vi "DB UI - Search-Load Setup.vi"(11 "Refnums":T4) -> (0 "Error Out":errorcluster, 1 "{Cancel}":bool, 2 "Transaction":T3, 3 "1D Results":string[](array[string]))   [LabVIEW 2013]
uses:
  Controls/Combo Box.ctl
  Controls/DB - Refnums.ctl
  Controls/Setup - Part Details - Item Details.ctl
  <vilib>/Utility/miscctls.llb/LVRectTypeDef.ctl
  Controls/Transaction Cluster.ctl
  Controls/Debug Tab.ctl
  <vilib>/Utility/miscctls.llb/LVRowAndColumnUnsignedTypeDef.ctl
  <vilib>/Utility/miscctls.llb/LVPointTypeDef.ctl
  <vilib>/Utility/miscctls.llb/LVRowAndColumnTypeDef.ctl
  Controls/DB - Setup Item Enum.ctl
panel:
  in  "OR [CaptionOnly]":string caption="OR"
  in  "Tab Control":T1
  out "Get Clicked Column Header":i32
  in  "Ascending":bool
  out "Time":u32
  out "x":u32
  out "y":u32
  out "Front Panel Window:Panel Bounds":T2
  out "2D Results":string[][](array[string])=[["Production", "OperationNo1"], ["Production", "Qty1"], ["Production", "NCRNo1"], ["Production", "CustomerID1"], ["Production", "Customer1"], ["Production", "Project1"], ["Production", "SalesOrderNo1"], ["Production", "SalesOrderItemNo1"], ["Production", "MaterialNo1"], ["Production", "MaterialRev1"], ["Production", "MaterialDesc1"], ["Production", "SerialNos1"], ["Production", "UnitOfQty1"]]
  out "Drop Down":bool
  in  "CellBG New Cells":u32(colorbox)=16777225
  in  "CellBG Unused Cells":u32(colorbox)=16777238
  in  "CellBG ColHdrs":u32(colorbox)=11776947
  out "MHandler Error":errorcluster
  in  "Criteria [CaptionOnly]":string caption="Criteria"
  in  "Cancel":bool caption="Report Execute Search"
  in  "Open":bool caption="Report Execute Search"
  in  "Search":bool caption="Report Execute Search"
  in  "Report List":i32(listbox)=-1 caption="List"
  in  "OrderNo":T5 caption="Order No."
  in  "TransactionNo":T5 caption="Transaction No."
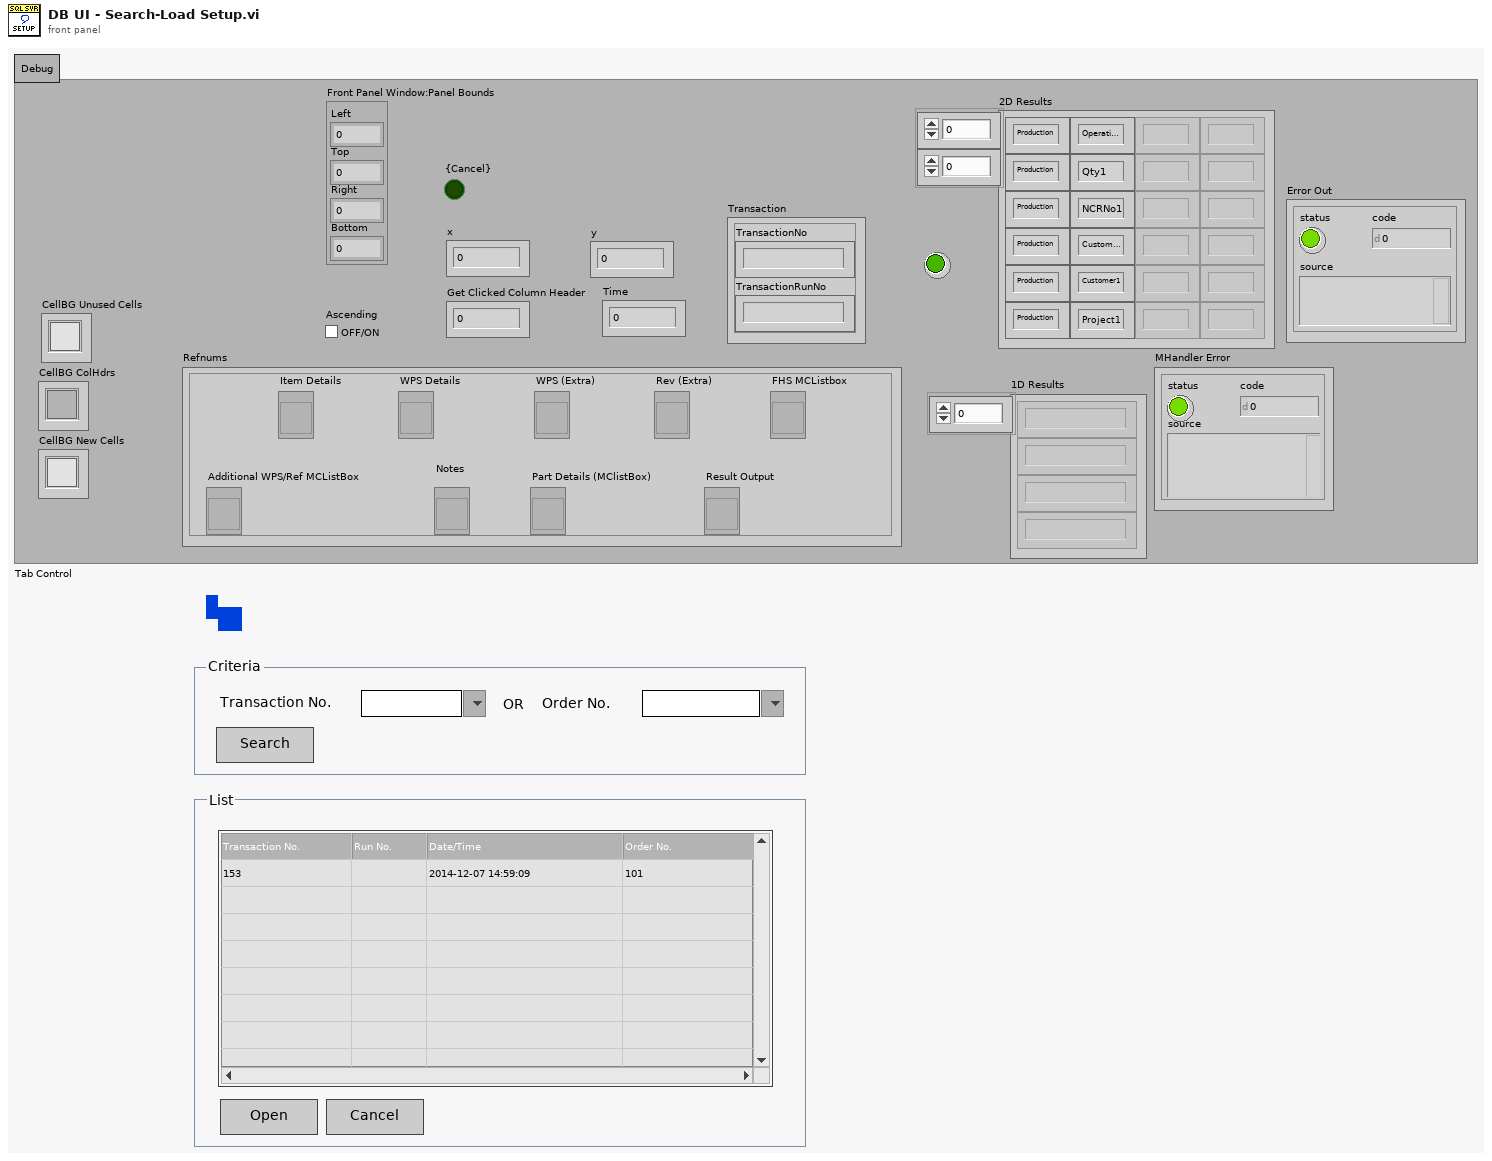
[diagram p1: front panel]
types:
  T1 = typedef "Debug Tab.ctl" = enum32{"Debug"}
  T2 = typedef "LVRectTypeDef.ctl" = cluster{"Left":i16, "Top":i16, "Right":i16, "Bottom":i16}
  T3 = typedef "Transaction Cluster.ctl" = cluster{"TransactionNo":string, "TransactionRunNo":string}
  T4 = typedef "DB - Refnums.ctl" = cluster{"Item Details":refnum<vi>, "WPS Details":refnum<vi>, "WPS (Extra)":refnum<vi>, "Rev (Extra) ":refnum<vi>, "FHS MCListbox":refnum<vi>, "Additional WPS/Ref MCListBox":refnum<vi>, "Notes":refnum<vi>, "Part Details (MClistBox)":refnum<vi>, "Result Output":refnum<vi>}
  T5 = typedef "Combo Box.ctl" = string
  T6 = typedef "LVPointTypeDef.ctl" = cluster{"Horizontal":i16, "Vertical":i16}
  T7 = typedef "LVRowAndColumnUnsignedTypeDef.ctl" = cluster{"Row":u32, "Column":u32}
  T8 = typedef "LVRowAndColumnTypeDef.ctl" = cluster{"Row":i32, "Column":i32}
  T9 = typedef "DB - Setup Item Enum.ctl" = enum16{"SELECT [Plant],[OrderNo]", "INSERT [Setup].[Header]", "INSERT [Setup].[Item]", "INSERT [Setup].[ProcedureItem]", "SELECT [TransactionNo]", "SELECT [TransactionNo], others", "SELECT [OrderNo]", "SELECT [OrderNo], others", "SELECT h.[TransactionNo], i.[OrderNo]", "SELECT [Setup].[ProcedureItem]", "SELECT [EquipmentxId]"}
  T10 = enum8{"Enabled", "Disabled", "Disabled and Grayed Out"}
  T11 = cluster{"TransactionNo":string, "TransactionRunNo":string}
  T12 = typedef "eventvkey.ctl" = enum16{"ASCII", "Enter", "Return", "Shift", "Ctrl", "Alt", "Cmd", "Opt", "Caps", "NumLock", "Clear", "Break", "Up", "Down", "Left", "Right", "Insert", "Delete", "Home", "End", "PageUp", "PageDown", "Escape", "Help", "Pause", "ScrollLock", "F1", "F2", "F3", "F4", "F5", "F6", "F7", "F8", "F9", "F10", "F11", "F12", "F13", "F14", "F15", "F16", "F17", "F18", "F19", "F20", "F21", "F22", "F23", "F24", "Play", "VolumeUp", "VolumeDown", "Mute", "Two Byte Char"}
  T13 = typedef "LVPoint32TypeDef.ctl" = cluster{"Horizontal":i32, "Vertical":i32}
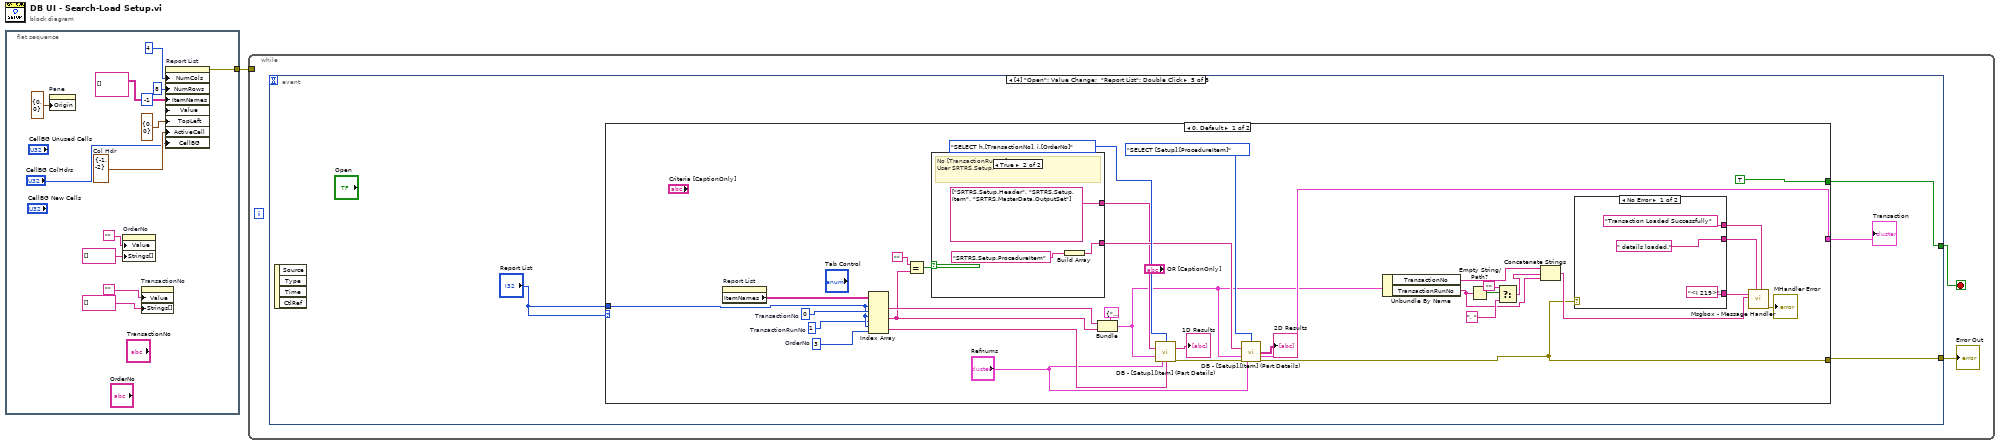
[diagram p0: block diagram]
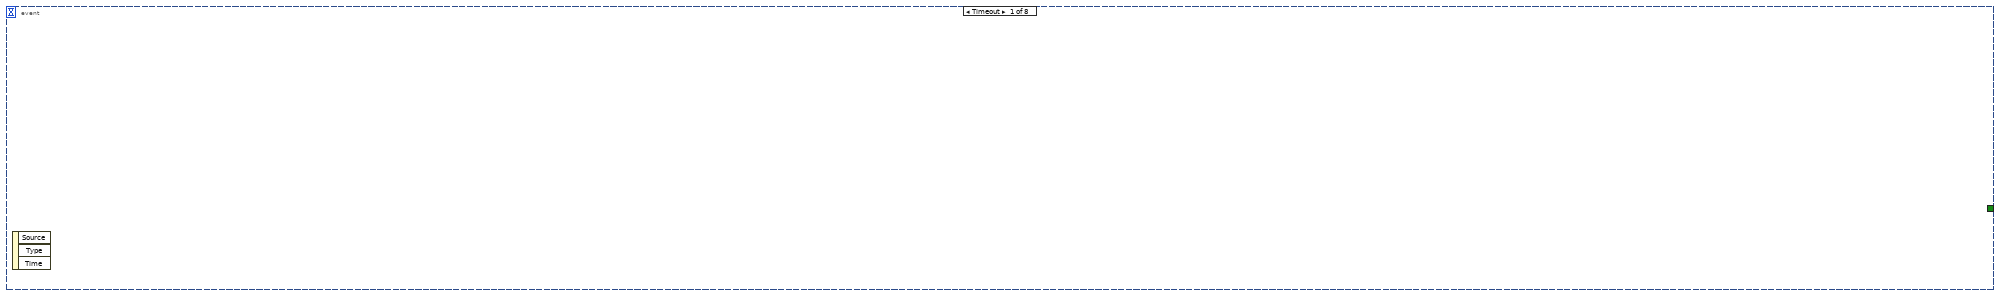
[diagram p2: hidden frame]
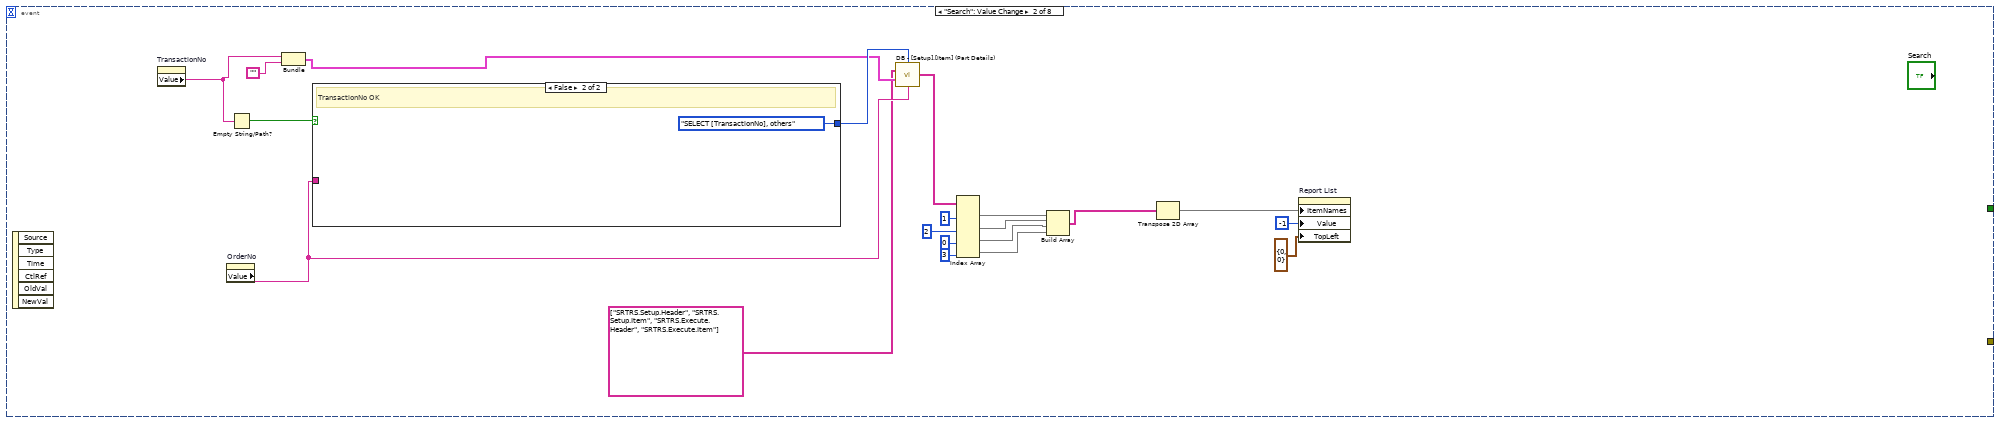
[diagram p3: hidden frame]
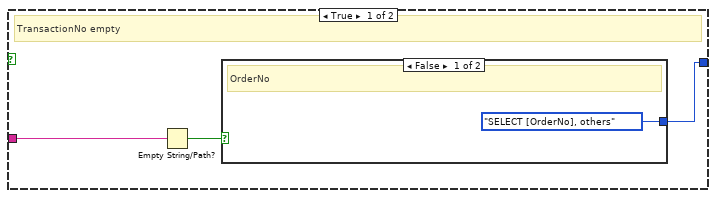
[diagram p4: hidden frame]
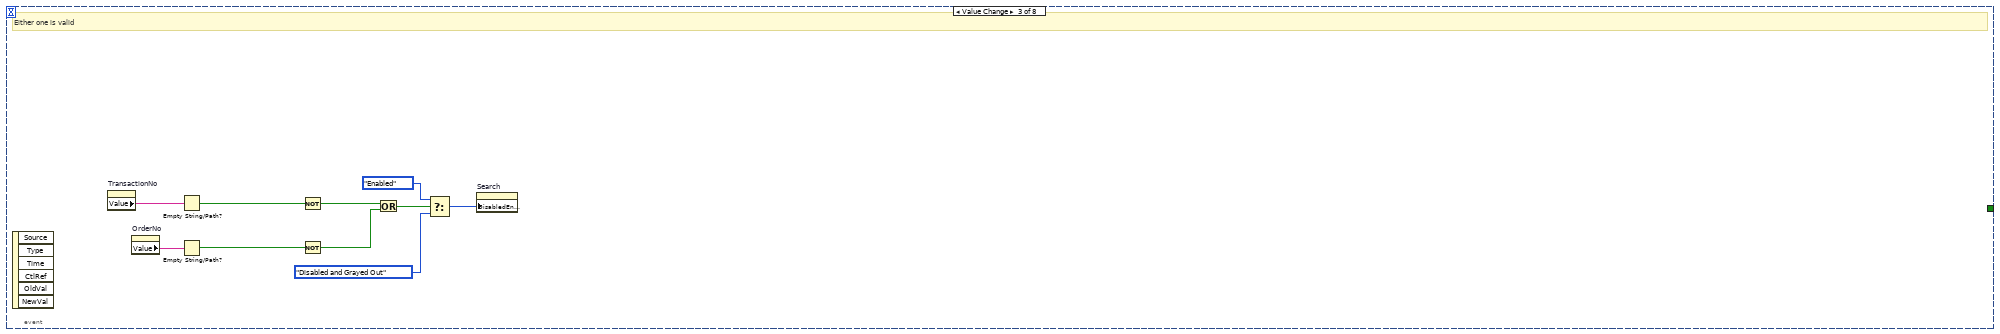
[diagram p6: hidden frame]
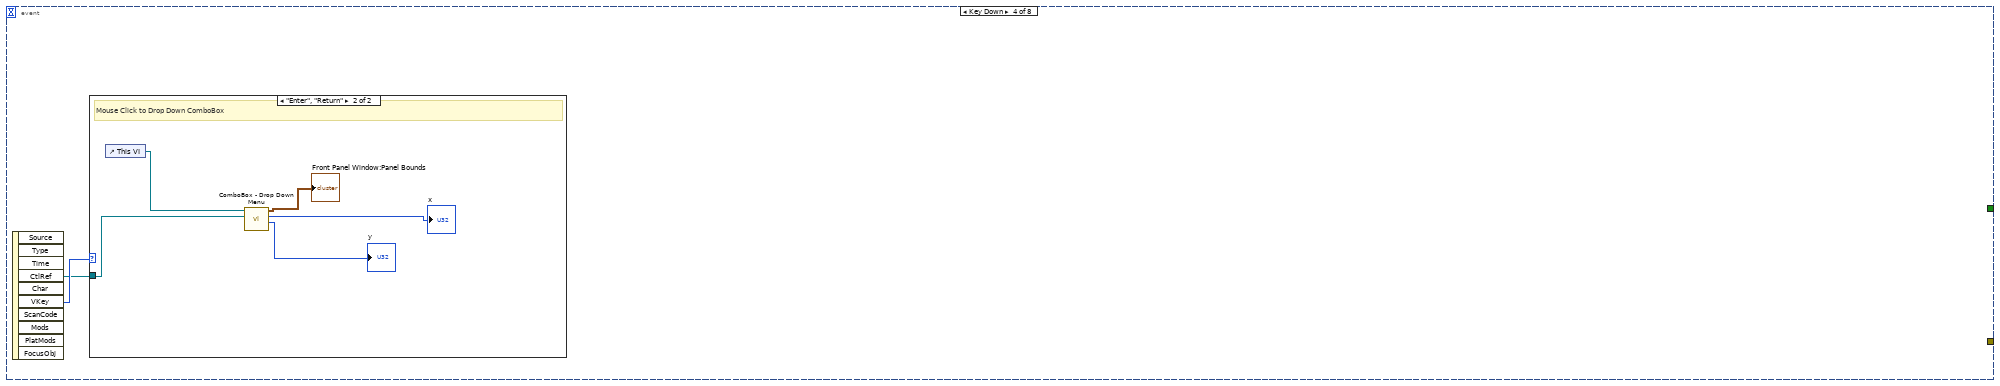
[diagram p7: hidden frame]
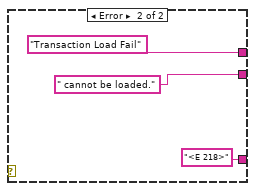
[diagram p9: hidden frame]
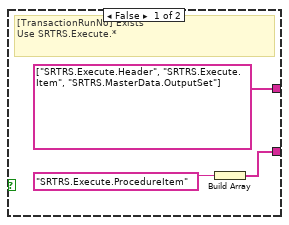
[diagram p10: hidden frame]
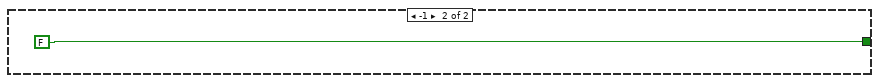
[diagram p11: hidden frame]
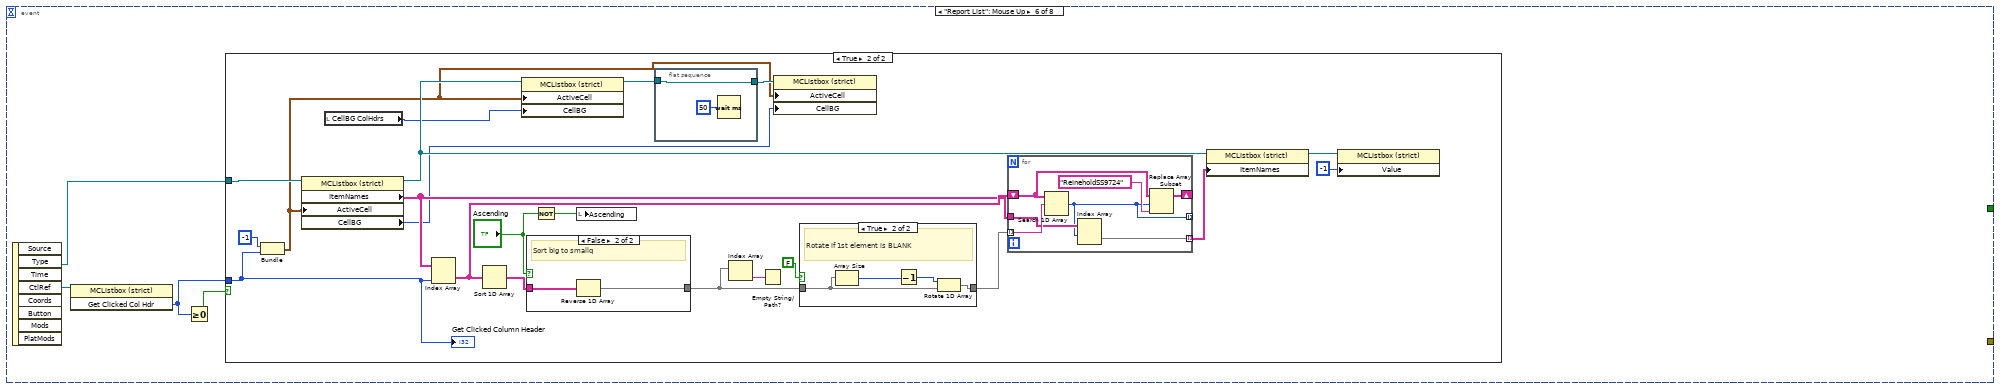
[diagram p12: hidden frame]
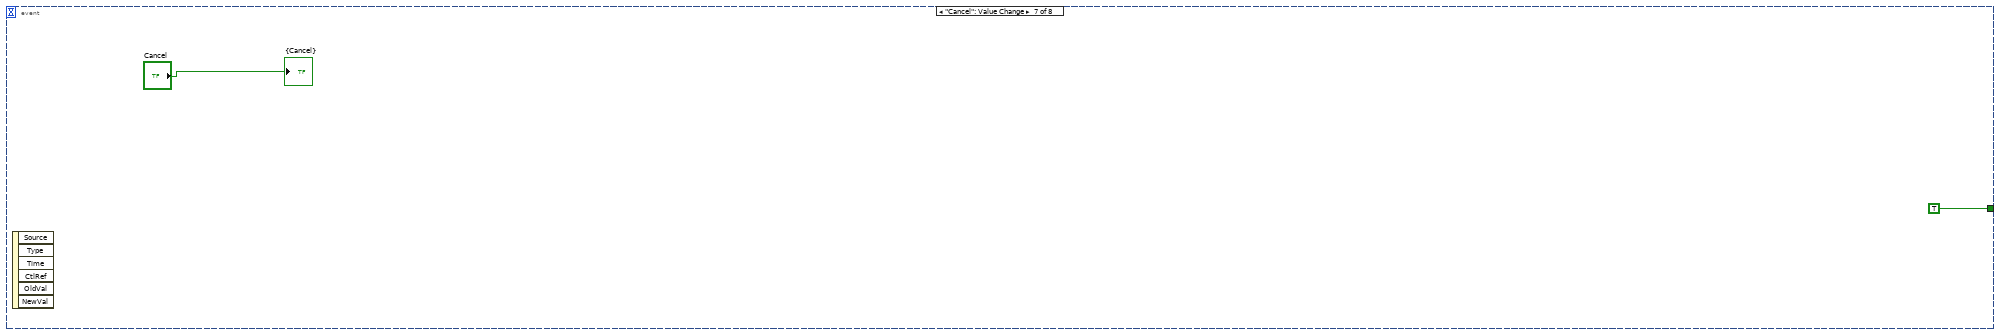
[diagram p16: hidden frame]
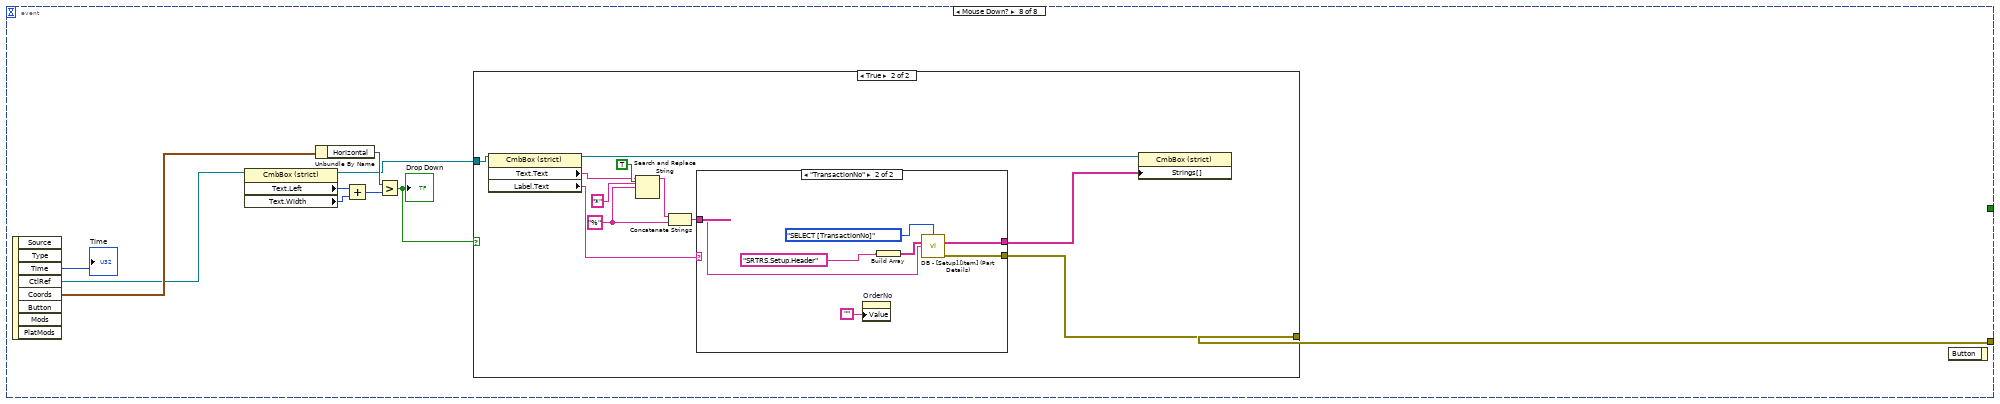
[diagram p17: hidden frame]
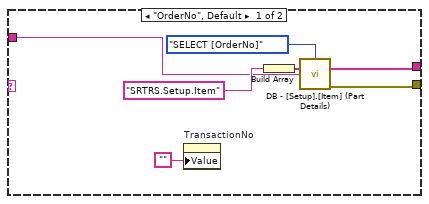
[diagram p19: hidden frame]
diagram:
  n1 = flat-sequence {
    tunnel: [w13] -> w1
    frame #0 {
      w3 = T8 {"Row"=-1, "Column"=-2}  # Col Hdr
      n2 = property on="Pane" class="Pane"("Origin"=T6 {"Horizontal"=0, "Vertical"=0}) -> ()  [unwired: 2 in, 2 out]
      n3 = property on="OrderNo" class="CmbBox (strict)"("Value"="", "Strings[]"=string[] [] ("Strings []")) -> ()  [unwired: 2 in, 2 out]
      n4 = property on="TransactionNo" class="CmbBox (strict)"("Value"="", "Strings[]"=string[] [] ("Strings []")) -> ()  [unwired: 2 in, 2 out]
      n5 = property on="Report List" class="MCListbox (strict)"("NumCols"=u32 4 ("Number of Columns"), "NumRows"=u32 8 ("Number of Rows"), "ItemNames"=string[][] [] ("Item Names"), "Value"=-1 ("Report List"), "TopLeft"=T7 {"Row"=0, "Column"=0} ("Top Left Visible Cell"), "ActiveCell"=w3, "CellBG"="CellBG ColHdrs") -> (error out=w13:errorcluster)  [unwired: 2 in, 1 out]
    }
  }
  n6 = while {
    tunnel: w1 -> [_]
    stop <- w16 stop-if-true
    n7 = event shown="[4] \"Open\": Value Change;  \"Report List\": Double Click" {
      selector: _ -> [_ _ _ _ _ _ _ _]
      dyn-events: _ -> [_ _ _ _ _ _ _ _]
      timeout: _ -> [_ _ _ _ _ _ _ _]
      tunnel: [_ _ _ _ w61 _ TRUE ("Cancel") _] -> w16
      tunnel: [_ _ _ _ w59 _ _ w162] -> w15
      event Timeout {
        n8 = event-data() -> ()  [unwired: 1 in, 3 out]
      }
      event "Search": Value Change {
        n9 = event-data() -> ()  [unwired: 1 in, 6 out]
        n10 = property on="TransactionNo" class="CmbBox (strict)"() -> ("Value"=w20:T5)  [unwired: 2 in, 2 out]
        n11 = property on="OrderNo" class="CmbBox (strict)"() -> ("Value"=w34:T5)  [unwired: 2 in, 2 out]
        n12 = Empty String/Path?(string/path=w20) -> (empty?=w36:bool)
        n13 = Bundle("Value"=w20, "") -> (w19:cluster{"Value":T5, string})  [unwired: 1 in]
        n14 = case shown="False" w36 {
          tunnel: w34 -> [w39 _]
          tunnel: [w37 DB_-_Setup_Item_Enum."SELECT [TransactionNo], others" ("DB - Setup Item Enum")] -> w35
          frame True {
            # "TransactionNo empty"
            n15 = Empty String/Path?(string/path=w39) -> (empty?=w38:bool)
            n16 = case shown="False" w38 {
              tunnel: [DB_-_Setup_Item_Enum."SELECT [OrderNo], others" ("DB - Setup Item Enum") _] -> w37
              frame False {
                # "OrderNo"
              }
              frame True {
                # "OrderNo empty"
              }
            }
          }
          frame False {
            # "TransactionNo OK"
          }
        }
        n17 = call "DB - [Setup].[Item] (Part Details).vi"("DB - Setup Item Enum"=w35, "DB.Schema.Table Array"=string[] ["SRTRS.Setup.Header", "SRTRS.Setup.Item", "SRTRS.Execute.Header", "SRTRS.Execute.Item"], "Transaction"=w19, "OrderNo"=w34) -> ("2D Results"=w31:string[][])  [unwired: 6 in, 5 out]
        n18 = Index Array(array=w31, index (col) #1=1 ("disabled index (col)"), index (col) #2=2 ("index (col)"), index (col) #3=0 ("index (col)"), index (col) #4=3 ("index (col)")) -> (element #1=w29:string[], element #2=w27:string[], element #3=w25:string[], element #4=w24:string[])  [unwired: 4 in]
        n19 = Build Array(w29, w27, w25, w24) -> (w23:string[][])
        n20 = Transpose 2D Array(2D array=w23) -> (transposed array=w22:string[][])
        n21 = property on="Report List" class="MCListbox (strict)"("ItemNames"=w22, "Value"=-1 ("Report List"), "TopLeft"=T7 {"Row"=0, "Column"=0} ("Top Left Visible Cell")) -> ()  [unwired: 2 in, 2 out]
      }
      event Value Change {
        # "Either one is valid"
        n22 = event-data() -> ()  [unwired: 1 in, 6 out]
        n23 = property on="TransactionNo" class="CmbBox (strict)"() -> ("Value"=w51:T5)  [unwired: 2 in, 2 out]
        n24 = property on="OrderNo" class="CmbBox (strict)"() -> ("Value"=w50:T5)  [unwired: 2 in, 2 out]
        n25 = Empty String/Path?(string/path=w51) -> (empty?=w49:bool)
        n26 = Empty String/Path?(string/path=w50) -> (empty?=w48:bool)
        n27 = Not(x=w49) -> (.not. x?=w47:bool)
        n28 = Not(x=w48) -> (.not. x?=w46:bool)
        n29 = Or(x=w47, y=w46) -> (x .or. y?=w45:bool)
        n30 = Select(t=T10."Enabled" ("Disabled"), s=w45, f=T10."Disabled and Grayed Out" ("Disabled")) -> (s? t:f=w43:T10)
        n31 = property on="Search" class="Bool"("DisabledEnum"=w43) -> ()  [unwired: 2 in, 2 out]
      }
      event Key Down {
        n32 = event-data() -> ("CtlRef"=w52:refnum<vi>, "VKey"=w53:T12)  [unwired: 1 in, 8 out]
        n33 = case shown="\"Enter\", \"Return\"" w53 {
          tunnel: w52 -> [_ w57]
          frame "ASCII", Default {
          }
          frame "Enter", "Return" {
            # "Mouse Click to Drop Down ComboBox"
            n34 = control-ref of="This VI"() -> (w58:refnum<vi>)
            n35 = call "ComboBox - Drop Down Menu.vi"("CtlRef"=w57, "VI in (This VI)"=w58) -> ("y"=→"y":u32, "x"=→"x":u32, "Front Panel Window:Panel Bounds"=→"Front Panel Window:Panel Bounds":T2)  [unwired: 7 in]
          }
        }
      }
      event "Open": Value Change; "Report List": Double Click {
        n36 = event-data() -> ()  [unwired: 1 in, 4 out]
        n37 = case shown="0, Default" "Report List" {
          tunnel: "Report List" -> [w86 _]
          tunnel: [w64 _] -> w59
          tunnel: [TRUE ("Cancel") FALSE ("Cancel")] -> w61
          tunnel: [w84 _] -> w60
          frame 0, Default {
            w85 = 1  # TransactionRunNo
            w88 = 3  # OrderNo
            w95 = 0  # TransactionNo
            n38 = property on="Report List" class="MCListbox (strict)"() -> ("ItemNames"=w96:string[][])  [unwired: 2 in, 2 out]
            n39 = Index Array(array=w96, index (row) #1=w86, index (col) #1=w95, index (row) #2=w86, index (col) #2=w85, index (row) #3=w86, index (col) #3=w88) -> (element #1=w89:string, element #2=w83:string, element #3=w87:string)
            n40 = Equal?(x="", y=w83) -> (x = y?=w81:bool)
            n41 = case shown="True" w81 {
              tunnel: [w104 w106] -> w79
              tunnel: [string[] ["SRTRS.Execute.Header", "SRTRS.Execute.Item", "SRTRS.MasterData.OutputSet"] string[] ["SRTRS.Setup.Header", "SRTRS.Setup.Item", "SRTRS.MasterData.OutputSet"]] -> w78
              frame False {
                # "[TransactionRunNo] Exists\nUse SRTRS.Execute.*"
                n42 = Build Array("SRTRS.Execute.ProcedureItem" ("DB.Schema.Table")) -> (w104:string[])
              }
              frame True {
                # "No [TransactionRunNo]\nUser SRTRS.Setup.*"
                n43 = Build Array("SRTRS.Setup.ProcedureItem" ("DB.Schema.Table")) -> (w106:string[])
              }
            }
            n44 = Bundle(cluster=T11 {"TransactionNo"="", "TransactionRunNo"=""} ("output cluster"), "TransactionNo"=w89, "TransactionRunNo"=w83) -> (w63:T11)
            n45 = call "DB - [Setup].[Item] (Part Details).vi"("DB - Setup Item Enum"=DB_-_Setup_Item_Enum."SELECT h.[TransactionNo], i.[OrderNo]", "DB.Schema.Table Array"=w78, "Transaction"=w63, "DB Refnums"="Refnums", "OrderNo"=w87) -> ("1D Results"=→"1D Results":string[], "SUMMARY"=w93:errorcluster)  [unwired: 5 in, 4 out]
            n46 = call "DB - [Setup].[Item] (Part Details).vi"("DB - Setup Item Enum"=DB_-_Setup_Item_Enum."SELECT [Setup].[ProcedureItem]", "DB.Schema.Table Array"=w79, "Transaction"=w63, "error in (no error)"=w93, "DB Refnums"="Refnums") -> ("2D Results"=→"2D Results":string[][], "Transaction"=w84:T3, "SUMMARY"=w64:errorcluster)  [unwired: 5 in, 3 out]
            n47 = Unbundle By Name(w63) -> ("TransactionNo"=w69:string, "TransactionRunNo"=w65:string)
            n48 = Empty String/Path?(string/path=w65) -> (empty?=w70:bool)
            n49 = Select(t="", s=w70, f=", ") -> (s? t:f=w66:string)
            n50 = Concatenate Strings(w69, w66, w65) -> (w72:string)
            n51 = case shown="No Error" w64 {
              tunnel: ["<I 219>" ("<.?....> Message Code") "<E 218>" ("<.?....> Message Code")] -> w75
              tunnel: ["Transaction Loaded Successfully" ("Short Description (When DB Not Available)") "Transaction Load Fail" ("Short Description (When DB Not Available)")] -> w74
              tunnel: [" details loaded." ("Description (When DB Not Available)") " cannot be loaded." ("Description (When DB Not Available)")] -> w73
              frame No Error {
              }
              frame Error {
              }
            }
            n52 = call "Msgbox - Message Handler.vi"("Short Description (When DB Not Available)"=w74, "Description (When DB Not Available)"=w73, "Pre-Description"=w72, "<.?....> Message Code"=w75) -> ("MHandler Error"=→"MHandler Error":errorcluster)  [unwired: 5 in, 2 out]
          }
          frame -1 {
          }
        }
        "Transaction" <- w60
      }
      event "Report List": Mouse Up {
        n53 = event-data() -> ("CtlRef"=w112:refnum<vi>)  [unwired: 1 in, 7 out]
        n54 = invoke class="MCListbox (strict)" method="Get Clicked Col Hdr"(reference=w112) -> ("Get Clicked Column Header"=w111:i32)  [unwired: 2 in, 2 out]
        n55 = Greater Or Equal To 0?(x=w111) -> (x >= 0?=w110:bool)
        n56 = case shown="True" w110 {
          tunnel: w112 -> [_ w126]
          tunnel: w111 -> [_ w119]
          frame False {
          }
          frame True {
            n57 = Bundle(-1, "Get Clicked Column Header"=w119) -> (w116:cluster{i32, "Get Clicked Column Header":i32})  [unwired: 1 in]
            n58 = property class="MCListbox (strict)"(reference=w126, "ActiveCell"=w116) -> (reference out=w121:refnum<vi>, "ItemNames"=w125:string[][], "CellBG"=w115:u32)  [unwired: 1 in, 1 out]
            n59 = local read "CellBG ColHdrs"() -> (w113:u32)
            n60 = Index Array(array=w125, index (col)=w119) -> (element=w129:string[])  [unwired: 1 in]
            n61 = Sort 1D Array(array=w129) -> (sorted array=w132:string[])
            n62 = property class="MCListbox (strict)"(reference=w121, "ActiveCell"=w116, "CellBG"=w113) -> (reference out=w118:refnum<vi>)  [unwired: 1 in, 1 out]
            n63 = case shown="False" "Ascending" {
              tunnel: w132 -> [w141 w143]
              tunnel: [w141 w142] -> w127
              frame True {
                # "Sort small to big p"
              }
              frame False {
                # "Sort big to smallq"
                n64 = Reverse 1D Array(array=w143) -> (reversed array=w142:string[])
              }
            }
            n65 = Not(x="Ascending") -> (.not. x?=w122:bool)
            n66 = local write "Ascending"(w122) -> ()
            n67 = flat-sequence {
              tunnel: w118 -> [w135]
              tunnel: [w135] -> w117
              frame #0 {
                n68 = Wait (ms)(milliseconds to wait=u32 50) -> ()  [unwired: 1 out]
              }
            }
            n69 = Index Array(array=w127) -> (element=w128:string)  [unwired: 1 in]
            n70 = Empty String/Path?(string/path=w128) -> ()  [unwired: 1 out]
            n71 = property class="MCListbox (strict)"(reference=w117, "ActiveCell"=w116, "CellBG"=w115) -> ()  [unwired: 1 in, 2 out]
            n72 = case shown="True" FALSE {
              tunnel: w127 -> [w136 w139]
              tunnel: [w136 w140] -> w124
              frame False {
              }
              frame True {
                # "Rotate if 1st element is BLANK"
                n73 = Array Size(array=w139) -> (size(s)=w138:i32)
                n74 = Decrement(x=w138) -> (x-1=w137:i32)
                n75 = Rotate 1D Array(1:w139, 2:w137) -> (0:w140:string[])
              }
            }
            n76 = for {
              tunnel: w124 -> [w150] mode=indexing
              shift-right: [w147] -> _
              shift-left: w129 -> [w149]
              tunnel: [w144] -> _ mode=indexing
              tunnel: w125 -> [w146]
              tunnel: [w145] -> w133 mode=indexing
              n77 = Search 1D Array(1D array=w149, element=w150) -> (index of element=w144:i32)  [unwired: 1 in]
              n78 = Index Array(array=w146, index (row)=w144) -> (element=w145:string[])  [unwired: 1 in]
              n79 = Replace Array Subset(array=w149, new element="ReineholdSS9724" ("new element/subarray"), index=w144) -> (w147:string[])
            }
            n80 = property class="MCListbox (strict)"(reference=w121, "ItemNames"=w133) -> (reference out=w131:refnum<vi>)  [unwired: 1 in, 1 out]
            n81 = property class="MCListbox (strict)"(reference=w131, "Value"=-1) -> ()  [unwired: 1 in, 2 out]
            "Get Clicked Column Header" <- w119
          }
        }
      }
      event "Cancel": Value Change {
        n82 = event-data() -> ()  [unwired: 1 in, 6 out]
        "{Cancel}" <- "Cancel"
      }
      event Mouse Down? {
        n83 = event-data() -> ("Time"=→"Time":u32, "CtlRef"=w155:refnum<vi>, "Coords"=w158:T13)  [unwired: 1 in, 5 out]
        n84 = property on="Property Node" class="CmbBox (strict)"(reference=w155) -> (reference out=w154:refnum<vi>, "Text.Left"=w160:i32, "Text.Width"=w159:u32)  [unwired: 1 in, 1 out]
        n85 = Unbundle By Name(w158) -> ("Horizontal"=w157:i32)
        n86 = Add(x=w160, y=w159) -> (x+y=w156:u32)
        n87 = Greater?(x=w157, y=w156) -> (0:w153:bool)
        "Drop Down" <- w153
        n88 = case shown="True" w153 {
          tunnel: [_ w173] -> w162
          tunnel: w154 -> [_ w167]
          frame False {
          }
          frame True {
            w168 = "%" ("replace string (\"\")")
            n89 = property on="Property Node" class="CmbBox (strict)"(reference=w167) -> (reference out=w165:refnum<vi>, "Text.Text"=w171:string, "Label.Text"=w163:string)  [unwired: 1 in, 1 out]
            n90 = Search and Replace String(replace all?=TRUE ("replace all? (F)"), input string=w171, search string="*", replace string=w168) -> (result string=w169:string)  [unwired: 4 in, 3 out]
            n91 = Concatenate Strings(w169, w168) -> (w164:string)
            n92 = case shown="\"TransactionNo\"" w163 {
              tunnel: [w177 w187] -> w173
              tunnel: [w179 w185] -> w166
              tunnel: w164 -> [w174 w181]
              frame "OrderNo", Default {
                n93 = property on="TransactionNo" class="CmbBox (strict)"("Value"="") -> ()  [unwired: 2 in, 2 out]
                n94 = Build Array("SRTRS.Setup.Item" ("DB.Schema.Table")) -> (w176:string[])
                n95 = call "DB - [Setup].[Item] (Part Details).vi"("DB - Setup Item Enum"=DB_-_Setup_Item_Enum."SELECT [OrderNo]", "DB.Schema.Table Array"=w176, "Search Parameters"=w174) -> ("1D Results"=w179:string[], "SUMMARY"=w177:errorcluster)  [unwired: 7 in, 4 out]
              }
              frame "TransactionNo" {
                n96 = property on="OrderNo" class="CmbBox (strict)"("Value"="") -> ()  [unwired: 2 in, 2 out]
                n97 = Build Array("SRTRS.Setup.Header" ("DB.Schema.Table")) -> (w183:string[])
                n98 = call "DB - [Setup].[Item] (Part Details).vi"("DB - Setup Item Enum"=DB_-_Setup_Item_Enum."SELECT [TransactionNo]", "DB.Schema.Table Array"=w183, "Search Parameters"=w181) -> ("1D Results"=w185:string[], "SUMMARY"=w187:errorcluster)  [unwired: 7 in, 4 out]
              }
            }
            n99 = property on="Property Node" class="CmbBox (strict)"(reference=w165, "Strings[]"=w166) -> ()  [unwired: 1 in, 2 out]
          }
        }
        n100 = event-data() -> ()  [unwired: 2 in, 1 out]
      }
    }
    "Error Out" <- w15
  }
